vi "recognize_script.vi"(1 "模板地址":path, 2 "识别数据特征":dbl[][](array[numeric]), 4 "选择感情数":i32) -> (8 "数值":dbl, 9 "结果":string)   [LabVIEW 2014]
panel:
  out "数值 4":dbl
  out "数值 2":dbl
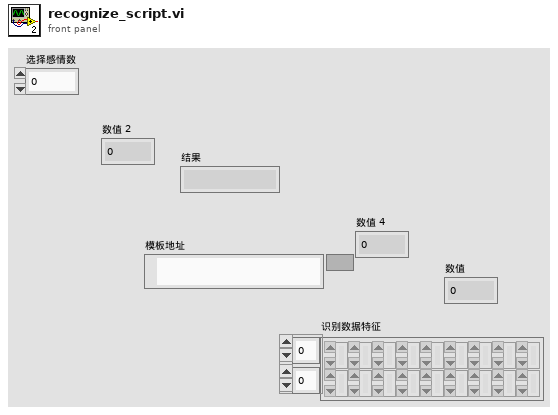
[diagram p1: front panel]
types:
  T1 = cluster{dbl[][], dbl[][], dbl[][], dbl[][], dbl[][], dbl[][], dbl[][], string, string, string, string}
  T2 = cluster{dbl[][], dbl[][], dbl[][], dbl[][], dbl[][], dbl[][], dbl[][], string, string, string, string, string}
  T3 = cluster{dbl[][], dbl[][], dbl[][], dbl[][], dbl[][], dbl[][], dbl[][], string, string, string, string, string, string}
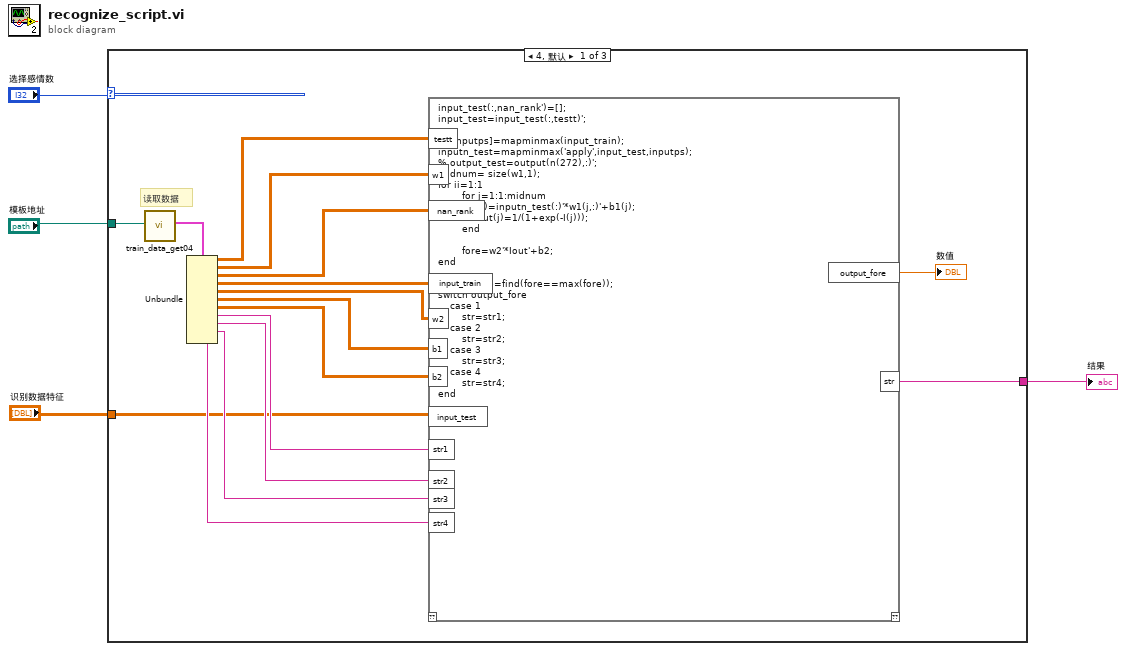
[diagram p0: block diagram]
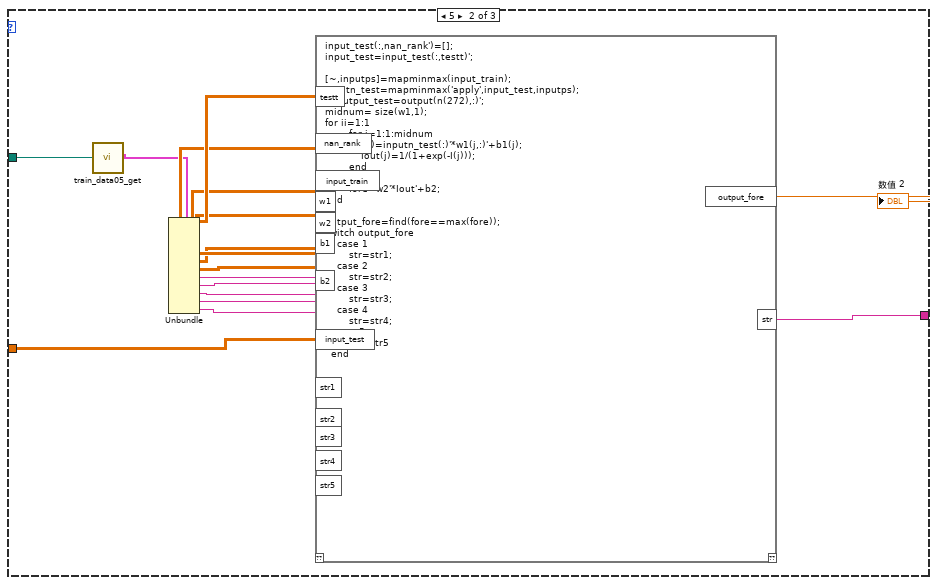
[diagram p2: hidden frame]
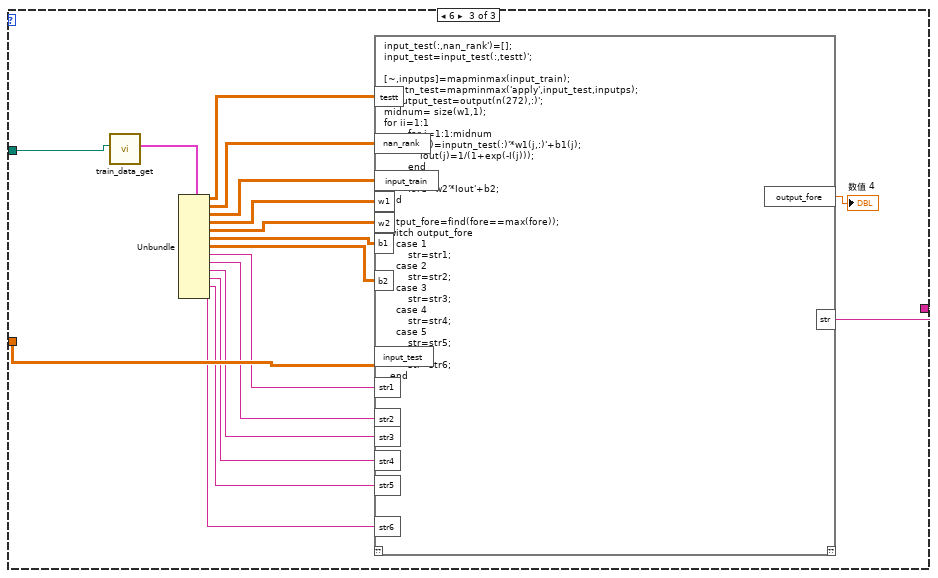
[diagram p3: hidden frame]
diagram:
  n1 = case shown="4, 默认" "选择感情数" {
    tunnel: "识别数据特征" -> [w12 w36 w54]
    tunnel: [w19 w35 w55] -> w2
    tunnel: "模板地址" -> [w18 w21 w53]
    frame 4, Default {
      # "读取数据"
      n2 = call "train_data_get04.vi"("文件路径（使用对话框）"=w18) -> ("数据"=w17:T1)  [unwired: 10 in]
      n3 = Unbundle(w17) -> (w6:dbl[][], w11:dbl[][], w7:dbl[][], w5:dbl[][], w10:dbl[][], w8:dbl[][], w9:dbl[][], w13:string, w14:string, w15:string, w16:string)
      n4 = script code="input_test(:,nan_rank')=[];\ninput_test=input_test(:,testt)';\n\n[~,inputps]=mapminmax(input_train);\ninputn_test=mapminmax('apply',input_test,inputps);\n% output_test=output(n(272),:)';\nmidnum= size(w1,1);\nfor ii=1:1\n        for j=1:1:midnum\n            I(j)=inputn_test(:)'*w1(j,:)'+b1(j);\n            Iout(j)=1/(1+exp(-I(j)));\n        end\n        \n        fore=w2'*Iout'+b2;\nend\n\noutput_fore=find(fore==max(fore));\nswitch output_fore\n    case 1\n        str=str1;\n    case 2\n        str=str2;\n    case 3\n        str=str3;\n    case 4\n        str=str4;\nend"("input_test"=w12, "testt"=w6, "nan_rank"=w7, "input_train"=w5, "b1"=w8, "w1"=w11, "b2"=w9, "w2"=w10, "str1"=w13, "str2"=w14, "str3"=w15, "str4"=w16) -> ("output_fore"=→"数值":dbl, "str"=w19:string)  [unwired: 1 in, 1 out]
    }
    frame 5 {
      n5 = call "train_data05_get.vi"("文件路径（使用对话框）"=w21) -> ("数据"=w22:T2)  [unwired: 10 in]
      n6 = Unbundle(w22) -> (w34:dbl[][], w33:dbl[][], w32:dbl[][], w31:dbl[][], w30:dbl[][], w29:dbl[][], w28:dbl[][], w27:string, w26:string, w25:string, w24:string, w23:string)
      n7 = script code="input_test(:,nan_rank')=[];\ninput_test=input_test(:,testt)';\n\n[~,inputps]=mapminmax(input_train);\ninputn_test=mapminmax('apply',input_test,inputps);\n% output_test=output(n(272),:)';\nmidnum= size(w1,1);\nfor ii=1:1\n        for j=1:1:midnum\n            I(j)=inputn_test(:)'*w1(j,:)'+b1(j);\n            Iout(j)=1/(1+exp(-I(j)));\n        end\n        \n        fore=w2'*Iout'+b2;\nend\n\noutput_fore=find(fore==max(fore));\nswitch output_fore\n    case 1\n        str=str1;\n    case 2\n        str=str2;\n    case 3\n        str=str3;\n    case 4\n        str=str4;\n   case 5\n        str=str5\n  end"("input_test"=w36, "testt"=w34, "nan_rank"=w33, "input_train"=w32, "b1"=w29, "w1"=w31, "b2"=w28, "w2"=w30, "str1"=w27, "str2"=w26, "str3"=w25, "str4"=w24, "str5"=w23) -> ("output_fore"=→"数值 2":dbl, "str"=w35:string)  [unwired: 1 in, 1 out]
    }
    frame 6 {
      n8 = call "train_data_get.vi"("文件路径（使用对话框）"=w53) -> ("数据 2"=w52:T3)  [unwired: 10 in]
      n9 = Unbundle(w52) -> (w51:dbl[][], w50:dbl[][], w49:dbl[][], w48:dbl[][], w47:dbl[][], w46:dbl[][], w45:dbl[][], w39:string, w40:string, w41:string, w42:string, w43:string, w44:string)
      n10 = script code="input_test(:,nan_rank')=[];\ninput_test=input_test(:,testt)';\n\n[~,inputps]=mapminmax(input_train);\ninputn_test=mapminmax('apply',input_test,inputps);\n% output_test=output(n(272),:)';\nmidnum= size(w1,1);\nfor ii=1:1\n        for j=1:1:midnum\n            I(j)=inputn_test(:)'*w1(j,:)'+b1(j);\n            Iout(j)=1/(1+exp(-I(j)));\n        end\n        \n        fore=w2'*Iout'+b2;\nend\n\noutput_fore=find(fore==max(fore));\nswitch output_fore\n    case 1\n        str=str1;\n    case 2\n        str=str2;\n    case 3\n        str=str3;\n    case 4\n        str=str4;\n    case 5\n        str=str5;\n    case 6 \n        str=str6;\n  end"("input_test"=w54, "testt"=w51, "nan_rank"=w50, "input_train"=w49, "b1"=w46, "w1"=w48, "b2"=w45, "w2"=w47, "str1"=w39, "str2"=w40, "str3"=w41, "str4"=w42, "str5"=w43, "str6"=w44) -> ("output_fore"=→"数值 4":dbl, "str"=w55:string)  [unwired: 1 in, 1 out]
    }
  }
  "结果" <- w2
